vi "Write_timeoutStatusNotifier.vi"(8 "error in (no error)":errorcluster, 10 "timeoutStatusNotifier":i32=100, 11 "TcpServer in":refnum<class "TcpServer.lvclass">) -> (0 "error out":errorcluster, 3 "TcpServer out":refnum<class "TcpServer.lvclass">)   [LabVIEW 2018]
doc: "Write the timeoutStatusNotifier in ms."
uses:
  TcpServer.lvclass
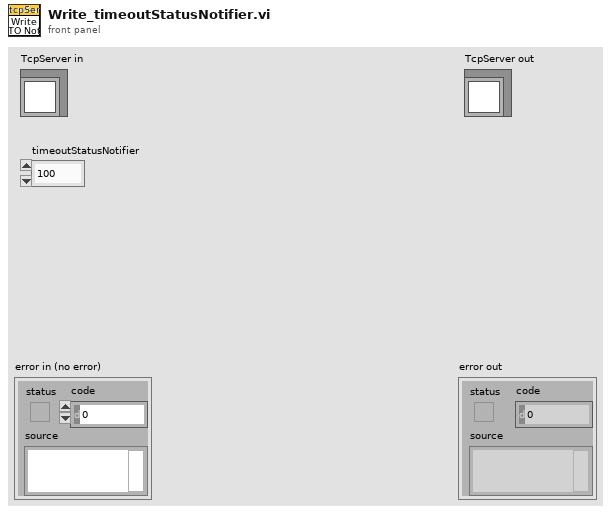
[diagram p1: front panel]
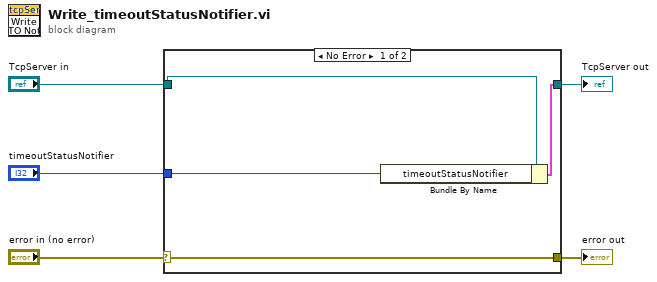
[diagram p0: block diagram]
diagram:
  n1 = case shown="No Error" "error in (no error)" {
    selector: "error in (no error)" -> [w9 w10]
    tunnel: [w9 w10] -> w4
    tunnel: [w7 w11] -> w2
    tunnel: "TcpServer in" -> [w8 w11]
    tunnel: "timeoutStatusNotifier" -> [w6 _]
    frame No Error {
      n2 = Bundle By Name(cluster=w8, "timeoutStatusNotifier"=w6) -> (w7:cluster{})
    }
    frame Error {
    }
  }
  "error out" <- w4
  "TcpServer out" <- w2
